vi "Read Input and Output Channel Count.vi"(8 "error in":errorcluster, 11 "Digital Input and Output Mode in":refnum<class "Digital Input and Output Mode.lvclass">) -> (0 "error out":errorcluster, 1 "Output Channels":i32, 2 "Input Channels":i32, 3 "Digital Input and Output Mode out":refnum<class "Digital Input and Output Mode.lvclass">)   [LabVIEW 2017, in "Scan Engine Scripting.lvlib" / "Digital Input and Output Mode.lvclass"]
uses:
  Digital Input and Output Mode.lvclass
  Digital Input and Output Mode.lvclass/Digital Input and Output Mode.ctl
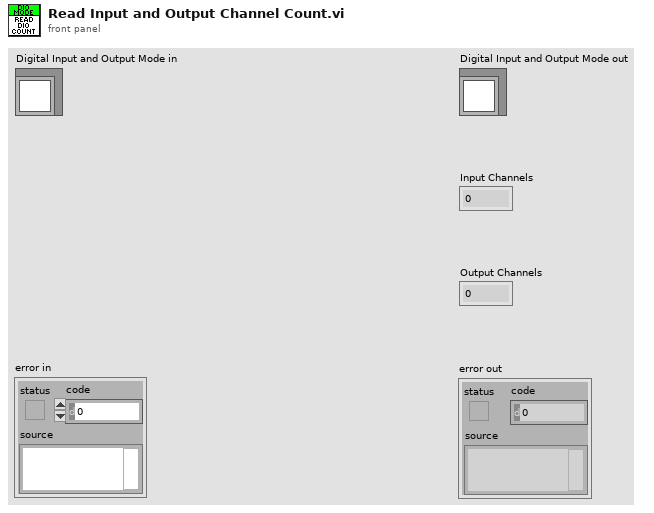
[diagram p1: front panel]
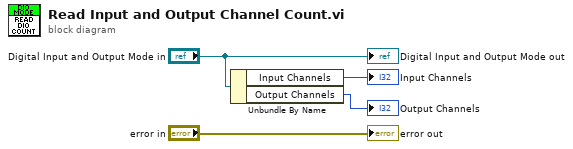
[diagram p0: block diagram]
diagram:
  n1 = Unbundle By Name("Digital Input and Output Mode in") -> ("Input Channels"=→"Input Channels":i32, "Output Channels"=→"Output Channels":i32)
  "error out" <- "error in"
  "Digital Input and Output Mode out" <- "Digital Input and Output Mode in"
